vi "NivelMedidodB.vi"(8 "error in (no error)":errorcluster, 10 "Voltaje":dbl, 11 "Prueba21 in":refnum<class "Prueba21.lvclass">) -> (0 "error out":errorcluster, 2 "Nivel Medido [dB]":dbl, 3 "Prueba21 out":refnum<class "Prueba21.lvclass">)   [LabVIEW 2019, in "Prueba21.lvclass"]
uses:
  Prueba21.lvclass
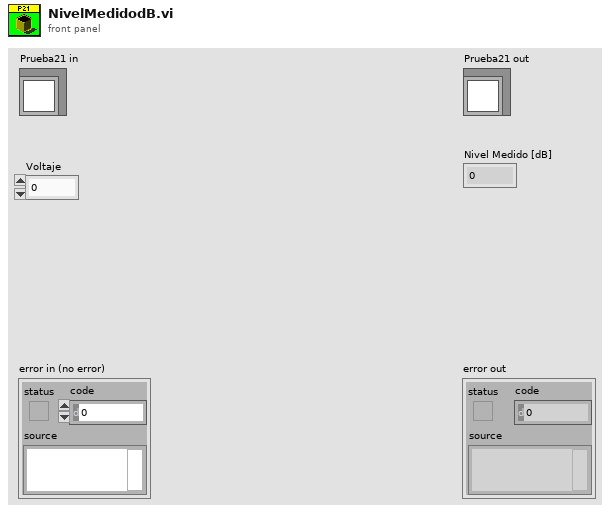
[diagram p1: front panel]
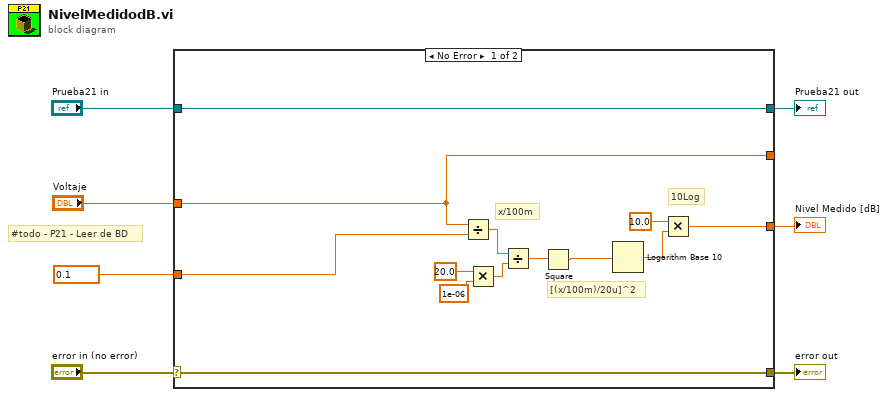
[diagram p0: block diagram]
diagram:
  w2 = 0.1 items=["10m"=0.01, "31,6m"=0.0316, "100m"=0.1, "316m"=0.316, "1"=1.0] ("Sensibilidad")
  # "#todo - P21 - Leer de BD"
  n1 = case shown="No Error" "error in (no error)" {
    selector: "error in (no error)" -> [w19 w22]
    tunnel: [w19 w22] -> w6
    tunnel: [w20 w21] -> w4
    tunnel: "Prueba21 in" -> [w20 w21]
    tunnel: "Voltaje" -> [w8 _]
    tunnel: w2 -> [w10 _]
    tunnel: [w8 _] -> _
    tunnel: [w9 _] -> w1
    frame No Error {
      # "10Log"
      # "[(x/100m)/20u]^2"
      # "x/100m"
      n2 = Divide(x=w8, y=w10) -> (x/y=w18:dbl)
      n3 = Multiply(x=20.0, y=1e-06) -> (x*y=w15:dbl)
      n4 = Divide(x=w18, y=w15) -> (x/y=w14:dbl)
      n5 = Square(x=w14) -> (x^2=w11:dbl)
      n6 = Logarithm Base 10(1:w11) -> (0:w12:dbl)
      n7 = Multiply(x=10.0, y=w12) -> (x*y=w9:dbl)
    }
    frame Error {
    }
  }
  "error out" <- w6
  "Prueba21 out" <- w4
  "Nivel Medido [dB]" <- w1
